vi "add data.vi"(8 "error in":errorcluster, 9 "Time Stamp (now: system time)":timestamp format="%<%x %.3X>T", 10 "Data Cluster":variant, 11 "stream custom cluster in":refnum<class "stream_custom_cluster.lvclass">) -> (0 "error out":errorcluster, 3 "stream custom cluster out":refnum<class "stream_custom_cluster.lvclass">)   [LabVIEW 2020, in "stream_custom_cluster.lvclass"]
doc: "Adds cluster data to the internal buffer for later transmission.\n<b>Data type must be identical to the Initialize function.</b>\nFast, non-blocking operation for high-speed data collection.\nSee `Streaming Cluster Data` example for useage notes."
uses:
  stream_custom_cluster.lvclass
  stream_custom_cluster.lvclass/stream_custom_cluster.ctl
  057b191d-3401-46d7-ac6b-70efd91a1f13.vi
  <vilib>/LabVIEW Open Source Project/Epoch Date & Time/epoch.UNIX/Epoch.UNIX.lvclass
  C:/Program Files/National Instruments/LabVIEW 2020/vi.lib/LabVIEW Open Source Project/Epoch Date & Time/epoch/Epoch.lvclass
  <vilib>/LabVIEW Open Source Project/Epoch Date & Time/Get Epoch Time.vi
  <vilib>/Utility/Data Type/Get Cluster Information.vi
  <vilib>/Utility/error.llb/Error Cluster From Error Code.vi
  <userlib>/_OpenG.lib/lvdata/lvdata.llb/openg_variant.lvlib
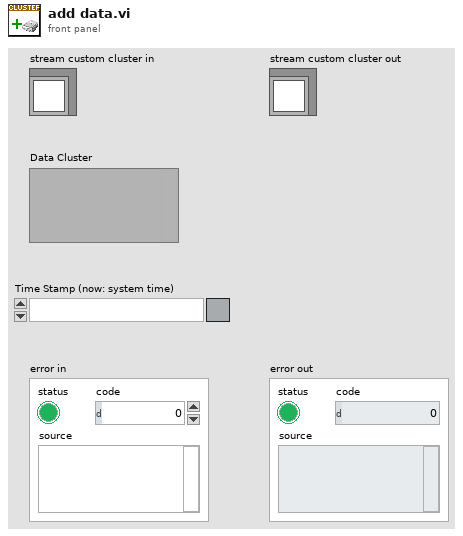
[diagram p1: front panel]
types:
  T1 = typedef "openg_variant.lvlib/Type Descriptor Enumeration__ogtk.ctl" = enum8{"<Null>", "I8", "I16", "I32", "I64", "U8", "U16", "U32", "U64", "SGL", "DBL", "EXT", "CSG", "CDB", "CXT", "0x0F", "0x10", "0x11", "0x12", "0x13", "0x14", "Enum U8", "Enum U16", "Enum U32", "Enum U64", "SGL PQ", "DBL PQ", "EXT PQ", "CSG PQ", "CDB PQ", "CXT PQ", "0x1F", "0x20", "Boolean", "0x22", "0x23", "0x24", "0x25", "0x26", "0x27", "0x28", "0x29", "0x2A", "0x2B", "0x2C", "0x2D", "0x2E", "0x2F", "String", "0x31", "Path", "Pict", "0x34", "0x35", "0x36", "DAQ", "0x38", "0x39", "0x3A", "0x3B", "0x3C", "0x3D", "0x3E", "0x3F", "Array", "0x41", "0x42", "0x43", "0x44", "0x45", "0x46", "0x47", "0x48", "0x49", "0x4A", "0x4B", "0x4C", "0x4D", "0x4E", "0x4F", "Cluster", "0x51", "0x52", "Variant", "Waveform", "0x55", "0x56", "0x57", "0x58", "0x59", "0x5A", "0x5B", "0x5C", "0x5D", "0x5E", "Fixed Point", "0x60", "0x61", "0x62", "0x63", "0x64", "0x65", "0x66", "0x67", "0x68", "0x69", "0x6A", "0x6B", "0x6C", "0x6D", "0x6E", "0x6F", "Refnum", "0x71", "0x72", "Set Collection", "Map Collection"}
  T2 = cluster{"UNIX Timestamp":cluster{"seconds":i32, "nanos":i32}, "Renamed Data":variant}
  T3 = typedef "stream_custom_cluster.lvclass/private data.ctl" = cluster{"type":T1[], "channel names":string[], "data":refnum<queue>[], "cluster element types":variant[]}
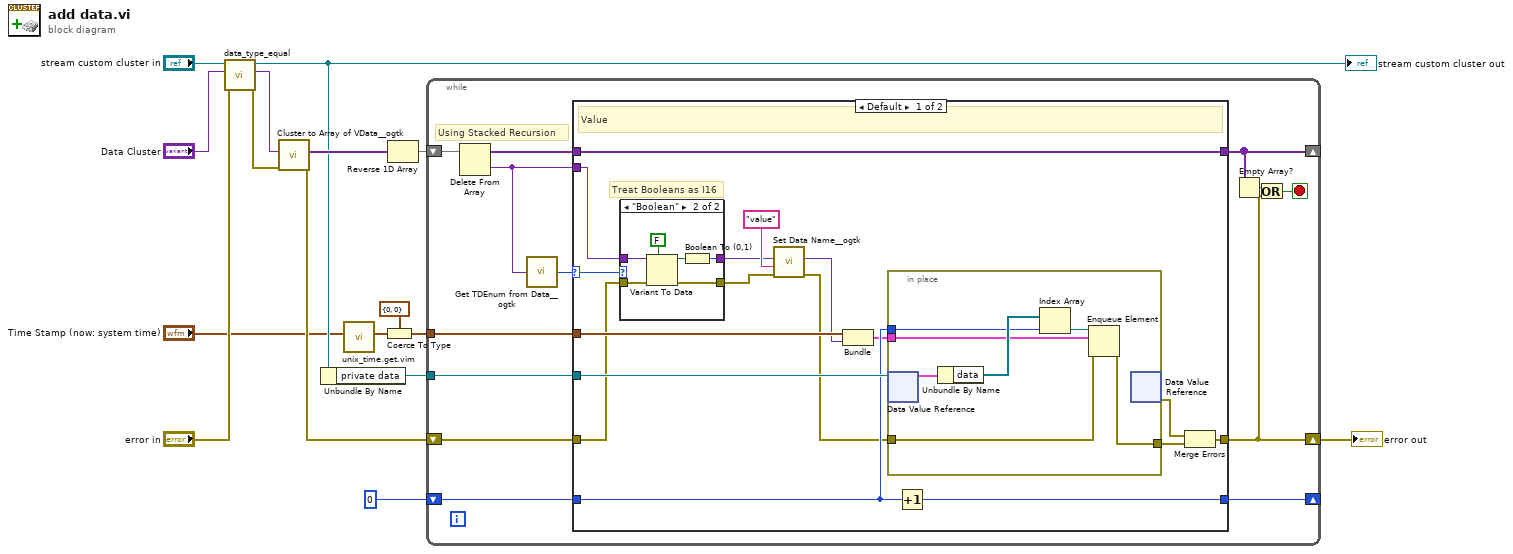
[diagram p0: block diagram]
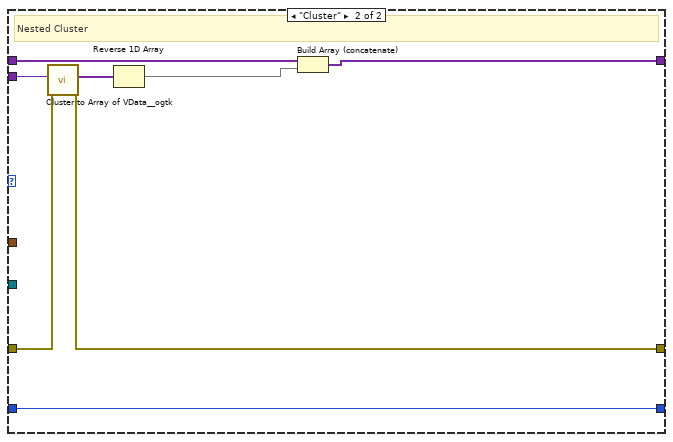
[diagram p3: hidden frame]
diagram:
  n1 = call "data_type_equal.vi"("error in"="error in", "Data Cluster"="Data Cluster", "Stream data cluster"="stream custom cluster in") -> ("error out"=w3:errorcluster, "dub Data Cluster"=w4:variant, "Stream data cluster out"=w6:refnum<class "stream_custom_cluster.lvclass">)  [unwired: 6 in]
  "stream custom cluster out" <- w6
  n2 = call <userlib>:"Cluster to Array of VData__ogtk.vi"("error in (no error)"=w3, "Cluster"=w4) -> ("error out"=w11:errorcluster, "Array of VData"=w16:variant[])  [unwired: 8 in]
  n3 = Unbundle By Name(w6) -> ("private data"=w9:refnum<data-value>)
  n4 = call "unix_time.get.vim"("Time Stamp (empty: now) [single or array]"="Time Stamp (now: system time)") -> ("UNIX Timestamp"=w13:cluster{"Seconds":i64, "Nanoseconds":i64})  [unwired: 10 in]
  n5 = Coerce To Type(0:w13, 1:cluster{"seconds":i32, "nanos":i32} {"seconds"=0, "nanos"=0} ("UNIX Timestamp")) -> (2:w12:cluster{"seconds":i32, "nanos":i32})
  n6 = Reverse 1D Array(array=w16) -> (reversed array=w15:variant[])
  n7 = while {
    shift-right: [w27] -> _
    shift-left: w15 -> [w29]
    tunnel: w12 -> [w24]
    shift-right: [w20] -> _
    shift-left: 0 -> [w19]
    tunnel: w9 -> [w18]
    shift-right: [w17] -> w8
    shift-left: w11 -> [w23]
    stop <- w25 stop-if-true
    # "Using Stacked Recursion"
    n8 = Delete From Array(array=w29) -> (deleted portion=w22:variant, array with subset deleted=w28:variant[])  [unwired: 2 in]
    n9 = call <userlib>:"Get TDEnum from Data__ogtk.vi"("Data"=w22) -> ("Type Descriptor Enumeration"=w21:T1)  [unwired: 4 in]
    n10 = case shown="Default" w21 {
      selector: w21 -> [w36 _]
      tunnel: w22 -> [w35 w66]
      tunnel: [w46 w67] -> w27
      tunnel: w28 -> [w46 w68]
      tunnel: [w38 w65] -> w17
      tunnel: w24 -> [w42 _]
      tunnel: w23 -> [w30 w63]
      tunnel: [w45 w62] -> w20
      tunnel: w19 -> [w43 w62]
      tunnel: w18 -> [w44 _]
      frame Default {
        # "Treat Booleans as I16"
        # "Value"
        n11 = case shown="\"Boolean\"" w36 {
          tunnel: w35 -> [w47 w54]
          tunnel: [w47 w51] -> w34
          tunnel: [w48 w50] -> w33
          tunnel: w30 -> [w48 w49]
          frame Default {
          }
          frame "Boolean" {
            n12 = Variant To Data(error in=w49, type=FALSE, Variant=w54) -> (data=w52:bool, error out=w50:errorcluster)
            n13 = Boolean To (0,1)(Boolean=w52) -> (0, 1=w51:i16)
          }
        }
        n14 = call <userlib>:"Set Data Name__ogtk.vi"("error in (no error)"=w33, "Data Name"="value", "Data"=w34) -> ("error out"=w32:errorcluster, "Renamed Data"=w31:variant)  [unwired: 7 in]
        n15 = Bundle("UNIX Timestamp"=w42, "Renamed Data"=w31) -> (w41:T2)  [unwired: 1 in]
        n16 = in-place {
          in-place-border: w43 -> [w59]
          in-place-border: w41 -> [w57]
          in-place-border: w32 -> [w56]
          in-place-border: [w55] -> w39
          n17 = in-place-dvr #1(w44) -> (w61:T3)  [unwired: 1 out]
          n18 = Unbundle By Name(w61) -> ("data"=w60:refnum<queue>[])
          n19 = Index Array(array=w60, index=w59) -> (element=w58:refnum<queue>)
          n20 = Enqueue Element(queue=w58, element=w57, error in (no error)=w56) -> (error out=w55:errorcluster)  [unwired: 1 in, 2 out]
          n21 = in-place-dvr #1() -> (w40:errorcluster)  [unwired: 1 in, 1 out]
        }
        n22 = Increment(x=w43) -> (x+1=w45:i32)
        n23 = Merge Errors(w40, w39) -> (w38:errorcluster)
      }
      frame "Cluster" {
        # "Nested Cluster"
        n24 = call <userlib>:"Cluster to Array of VData__ogtk.vi"("error in (no error)"=w63, "Cluster"=w66) -> ("error out"=w65:errorcluster, "Array of VData"=w64:variant[])  [unwired: 8 in]
        n25 = Reverse 1D Array(array=w64) -> (reversed array=w69:variant[])
        n26 = Build Array (concatenate)(w68, w69) -> (w67:variant[])
      }
    }
    n27 = Empty Array?(array=w27) -> (empty?=w26:bool)
    n28 = Or(x=w26, y=w17) -> (x .or. y?=w25:bool)
  }
  "error out" <- w8
